vi "Read Moves List Notifier.vi"(8 "error in (no error)":errorcluster, 11 "Burrow in":refnum<class "Burrow.lvclass">) -> (0 "error out":errorcluster, 2 "Moves List Notifier":refnum<notifier>, 3 "Burrow out":refnum<class "Burrow.lvclass">)   [LabVIEW 2019, in "23.lvlib" / "Burrow.lvclass"]
uses:
  Burrow.lvclass
  Burrow.lvclass/Burrow.ctl
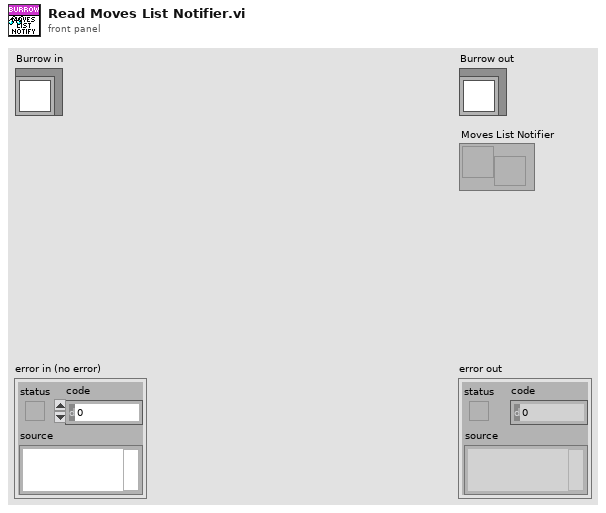
[diagram p1: front panel]
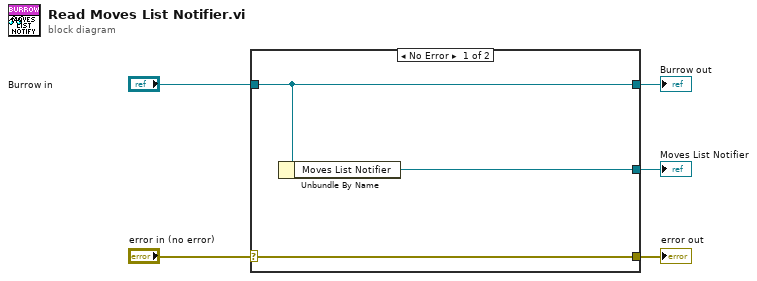
[diagram p0: block diagram]
diagram:
  n1 = case shown="No Error" "error in (no error)" {
    selector: "error in (no error)" -> [w8 w9]
    tunnel: [w8 w9] -> w4
    tunnel: [w7 w10] -> w2
    tunnel: "Burrow in" -> [w7 w10]
    tunnel: [w6 _] -> w1
    frame No Error {
      n2 = Unbundle By Name(w7) -> ("Moves List Notifier"=w6:refnum<notifier>)
    }
    frame Error {
    }
  }
  "error out" <- w4
  "Burrow out" <- w2
  "Moves List Notifier" <- w1
